vi "LSX Get Encoder.vi"(0 "lLSID":i32, 1 "pdRP":dbl, 5 "pdXP":dbl, 7 "pdYP":dbl, 9 "pdZP":dbl, 11 "error in (no error)":errorcluster) -> (3 "pdRP out":dbl, 4 "function return":i32, 6 "pdXP out":dbl, 8 "pdYP out":dbl, 10 "pdZP out":dbl, 15 "error out":errorcluster)   [LabVIEW 2016, in "Tango_DLL.lvlib"]
doc: "TANGOAPI int TANGOCALL LSX_GetEncoder (int lLSID, double *pdXP, double *pdYP, double *pdZP, double *pdRP);"
uses:
  Tango_DLL.lvlib
  2017/Microscope Control/Device Library/Stages/Marzhauser/SCAN IM 120 x 80/Tango DLL VIs/Tango_DLL.dll
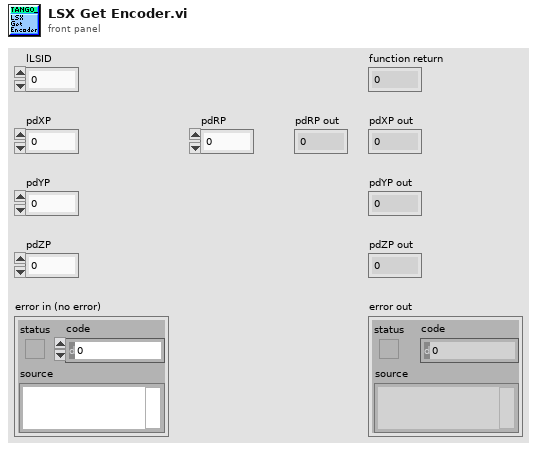
[diagram p1: front panel]
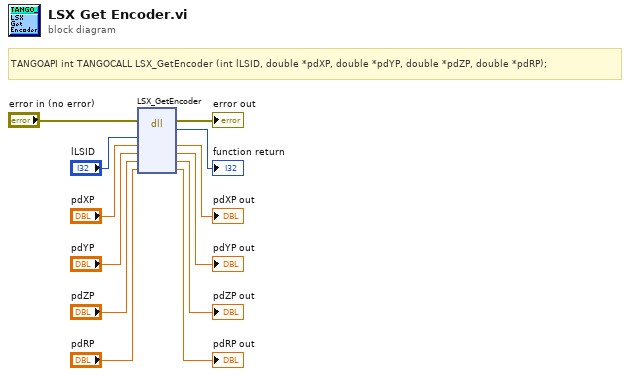
[diagram p0: block diagram]
diagram:
  # "TANGOAPI int TANGOCALL LSX_GetEncoder (int lLSID, double *pdXP, double *pdYP, double *pdZP, double *pdRP);"
  n1 = dll-call lib="C:/Users/4PiSMS/Documents/Microscope Control/2017/Microscope Control/Device Library/Stages/Marzhauser/SCAN IM 120 x 80/Tango DLL VIs/Tango_DLL.*" fn="LSX_GetEncoder"(error in="error in (no error)", "lLSID"="lLSID", "pdXP"="pdXP", "pdYP"="pdYP", "pdZP"="pdZP", "pdRP"="pdRP") -> (error out=→"error out":errorcluster, →"function return":i32, "pdXP"=→"pdXP out":dbl, "pdYP"=→"pdYP out":dbl, "pdZP"=→"pdZP out":dbl, "pdRP"=→"pdRP out":dbl)  [unwired: 3 in, 1 out]
